vi "ExampleServiceLabviewClient.vi"() -> ()   [LabVIEW 2011]
uses:
  C:/Users/wasonj/Documents/CATS/RobotRaconteur/RobotRaconteur/LabView/lvexamplethunk.dll
  lvexamplethunk.dll
panel:
  out "do_something":dbl
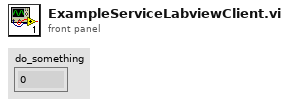
[diagram p1: front panel]
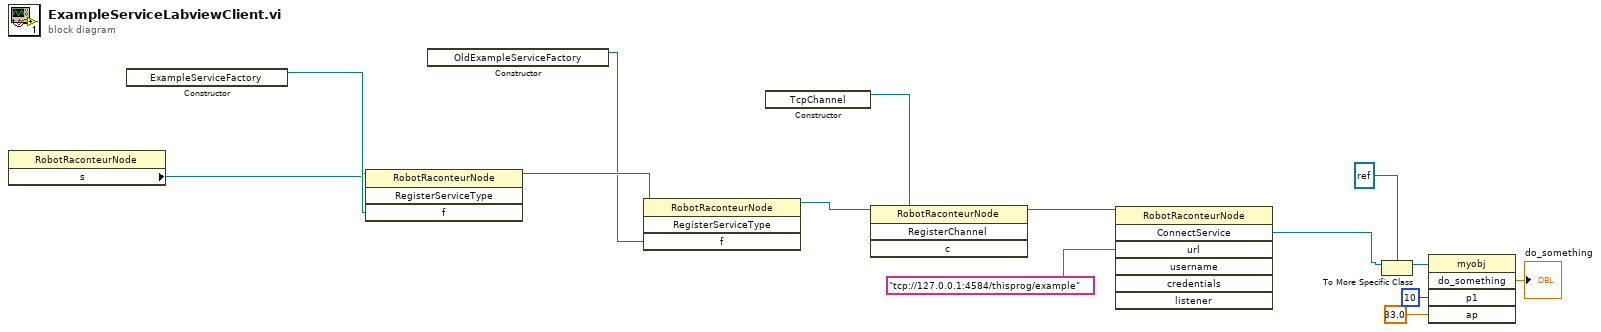
[diagram p0: block diagram]
diagram:
  n1 = property class="RobotRaconteurNode"() -> ("s"=w7:refnum<k24>)  [unwired: 2 in, 2 out]
  n2 = constructor class="ExampleServiceFactory"() -> (reference out=w13:refnum<k24>)  [unwired: 3 in, 2 out]
  n3 = invoke class="RobotRaconteurNode" method="RegisterServiceType"(reference=w7, "f"=w13) -> (reference out=w14:refnum<k24>)  [unwired: 2 in, 3 out]
  n4 = constructor class="OldExampleServiceFactory"() -> (reference out=w12:refnum<k24>)  [unwired: 3 in, 2 out]
  n5 = invoke class="RobotRaconteurNode" method="RegisterServiceType"(reference=w14, "f"=w12) -> (reference out=w11:refnum<k24>)  [unwired: 2 in, 3 out]
  n6 = constructor class="TcpChannel"() -> (reference out=w10:refnum<k24>)  [unwired: 3 in, 2 out]
  n7 = invoke class="RobotRaconteurNode" method="RegisterChannel"(reference=w11, "c"=w10) -> (reference out=w9:refnum<k24>)  [unwired: 2 in, 3 out]
  n8 = invoke class="RobotRaconteurNode" method="ConnectService"(reference=w9, "url"="tcp://127.0.0.1:4584/thisprog/example") -> ("ConnectService"=w6:refnum<k24>)  [unwired: 5 in, 6 out]
  n9 = To More Specific Class(target class=refnum<k24> refnum, reference=w6) -> (specific class reference=w4:refnum<k24>)  [unwired: 1 in, 1 out]
  n10 = invoke class="myobj" method="do_something"(reference=w4, "p1"=u16 10, "ap"=33.0) -> ("do_something"=→"do_something":dbl)  [unwired: 2 in, 4 out]
